vi "_Read.vi"(8 "error in (no error)":errorcluster, 11 "Temperature Controller.lvclass":refnum<class "Temperature Controller.lvclass">) -> (0 "error out":errorcluster, 2 "Data Points":dbl[](array[numeric]), 3 "Temperature Controller out":refnum<class "Temperature Controller.lvclass">)   [LabVIEW 2015, in "Temperature Controller.lvclass"]
uses:
  Temperature Controller.lvclass
  Temperature Controller.lvclass/Temperature Controller.ctl
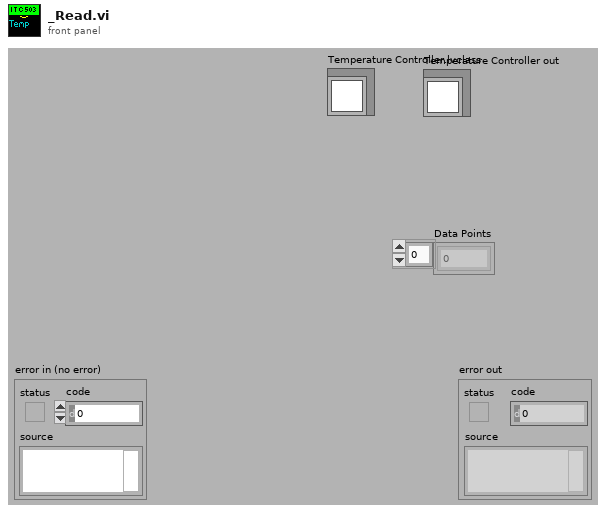
[diagram p1: front panel]
types:
  T1 = typedef "ITCIO.ctl" = cluster{"Address":T2, "Version":T3, "Ch 1 dec places":i16, "Ch 2 dec places":i16, "Ch 3 dec places":i16, "Ch1 Name":string, "Ch2 Name":string, "Ch3 Name":string}
  T2 = typedef "OxfordAddress.ctl" = cluster{"Com Port":i32, "ISOBUS Address":i32, "GPIB Address":i16, "Communication":enum16{"RS232", "ISOBUS", "GPIB", "Gateway"}}
  T3 = typedef "ITCVersion.ctl" = enum16{"ITC502", "ITC503", "ITC601"}
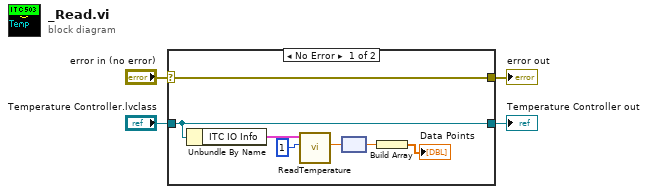
[diagram p0: block diagram]
diagram:
  n1 = case shown="No Error" "error in (no error)" {
    selector: "error in (no error)" -> [w7 w12]
    tunnel: [w7 w12] -> w3
    tunnel: [w6 w13] -> w2
    tunnel: "Temperature Controller.lvclass" -> [w6 w13]
    frame No Error {
      n2 = Unbundle By Name(w6) -> ("ITC IO Info"=w5:T1)
      n3 = call "ReadTemperature.vi"("Channel"=1, "IO Info"=w5) -> ("Temperature"=w10:dbl[unit])  [unwired: 5 out]
      n4 = node(w10) -> (w9:dbl)
      n5 = Build Array(w9) -> (→"Data Points":dbl[])
    }
    frame Error {
    }
  }
  "Temperature Controller out" <- w2
  "error out" <- w3
